vi "Cmd Get ADO Command Reference.vi"(4 "error in (no error)":errorcluster, 7 "command reference":T1) -> (0 "error out":errorcluster, 2 "ADODB._Command":refnum<k7>, 3 "command reference out":T1)   [LabVIEW 2020, in "NI_Database_API.lvlib"]
doc: "Returns the Command object refnum give the command reference."
uses:
  <vilib>/addons/database/NI_Database_API.lvlib
  <vilib>/addons/database/Command.llb/Cmd ObjectReference.ctl
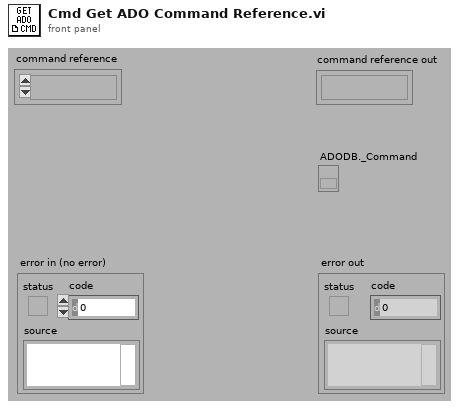
[diagram p1: front panel]
types:
  T1 = typedef "NI_Database_API.lvlib/Cmd ObjectReference.ctl" = refnum<k1>
  T2 = typedef "NI_Database_API.lvlib/Cmd DataMembers.ctl" = cluster{"ADODB._Command":refnum<k7>, "Connection":T3}
  T3 = typedef "NI_Database_API.lvlib/Conn ObjectReference.ctl" = refnum<k1>
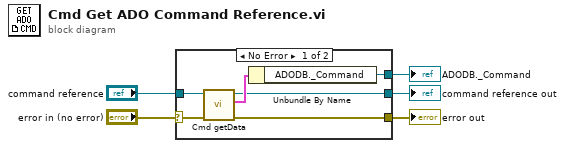
[diagram p0: block diagram]
diagram:
  n1 = case shown="No Error" "error in (no error)" {
    selector: "error in (no error)" -> [w6 w13]
    tunnel: [w11 _] -> w5
    tunnel: "command reference" -> [w10 w12]
    tunnel: [w8 w12] -> w3
    tunnel: [w7 w13] -> w2
    frame No Error {
      n2 = call <vilib>:"Cmd getData.vi"("error in (no error)"=w6, "command reference"=w10) -> ("error out"=w7:errorcluster, "data"=w9:T2, "command reference out"=w8:T1)  [unwired: 2 in, 1 out]
      n3 = Unbundle By Name(w9) -> ("ADODB._Command"=w11:refnum<k7>)
    }
    frame Error {
    }
  }
  "command reference out" <- w3
  "error out" <- w2
  "ADODB._Command" <- w5
